vi "ACTION.vi"(8 "error in (no error)":errorcluster, 9 "STEP State":T1, 10 "CORE":refnum<queue>, 11 "Mastering in":refnum<class "Mastering.lvclass">) -> (0 "error out":errorcluster, 3 "Mastering out":refnum<class "Mastering.lvclass">)   [LabVIEW 2014, in "SeqLoop.lvlib" / "STEP Classes.lvlib" / "Mastering.lvclass"]
uses:
  Mastering.lvclass
  TypeDefs/STEP State.ctl
  APIs/Message Queue/Message Cluster.ctl
  Mastering.lvclass/Mastering.ctl
  APIs/Message Queue/Enqueue Message (Array).vi
  APIs/Message Queue/Enqueue Message (Single).vi
  APIs/Message Queue/WINFAS 2 Message Queue.lvlib
  SeqLoop.lvlib
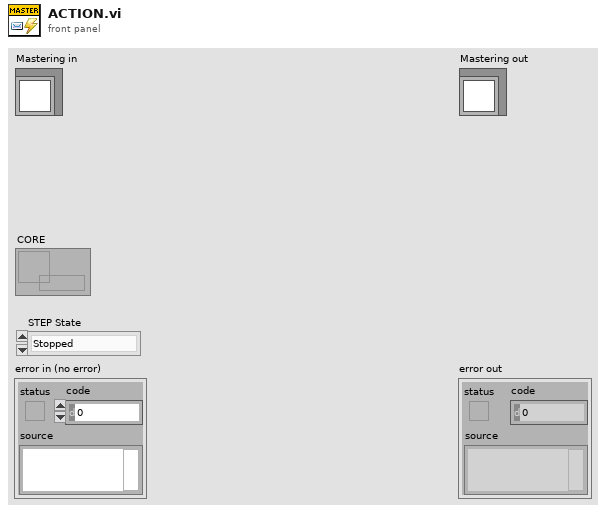
[diagram p1: front panel]
types:
  T1 = typedef "SeqLoop.lvlib/STEP State.ctl" = enum16{"Stopped", "First Call", "Idle...", "Advance OK", "Alarm", "Output Security", "Error"}
  T2 = cluster{"HWSync 1":bool, "HWSync 2":bool, "HWSync 3":bool, "HWSync 4":bool, "HWSync 5":bool}
  T3 = cluster{"MAX(T) or MIN (F)?":bool, "Mastering TDX Index":i32[]}
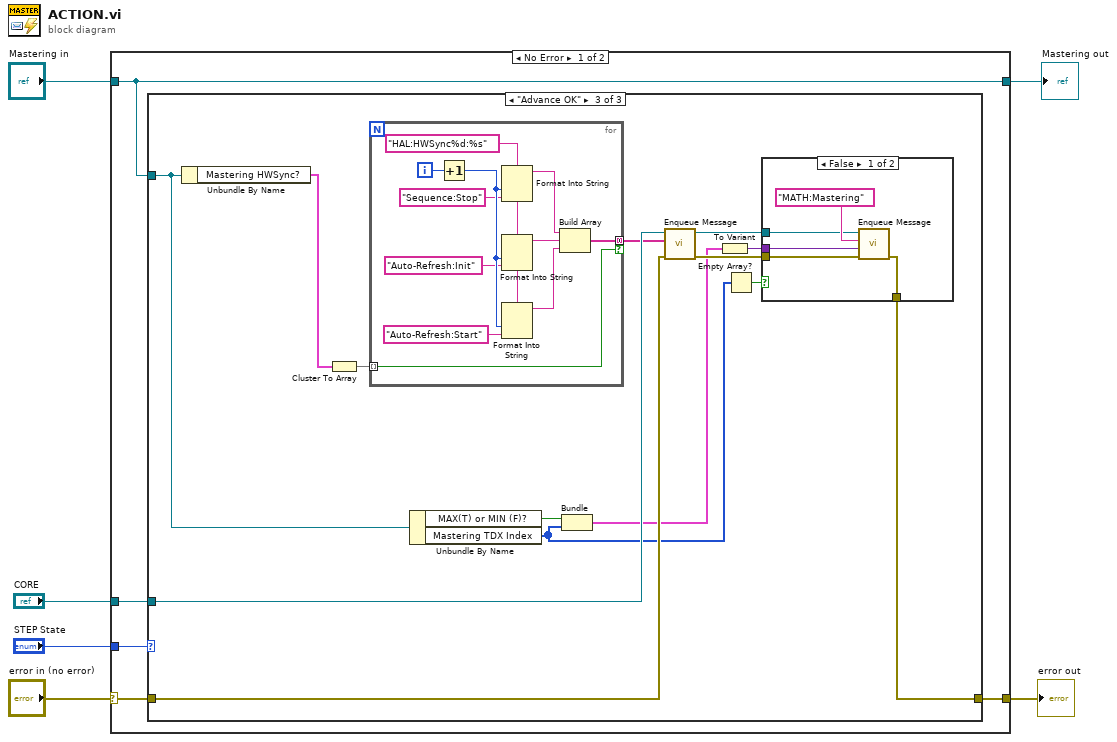
[diagram p0: block diagram]
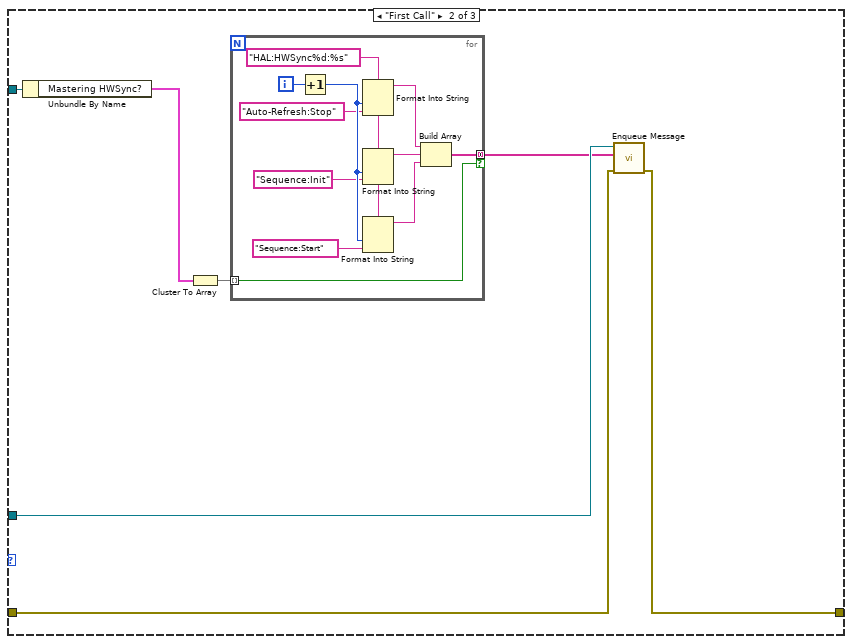
[diagram p3: hidden frame]
diagram:
  n1 = case shown="No Error" "error in (no error)" {
    selector: "error in (no error)" -> [w8 w63]
    tunnel: [w7 w63] -> w2
    tunnel: [w9 w62] -> w1
    tunnel: "Mastering in" -> [w9 w62]
    tunnel: "CORE" -> [w10 _]
    tunnel: "STEP State" -> [w11 _]
    frame No Error {
      n2 = case shown="\"Advance OK\"" w11 {
        tunnel: w10 -> [_ w16 w42]
        tunnel: w9 -> [_ w18 w37]
        tunnel: w8 -> [w12 w15 w41]
        tunnel: [w12 w14 w38] -> w7
        frame Default {
        }
        frame "First Call" {
          n3 = Unbundle By Name(w18) -> ("Mastering HWSync?"=w17:T2)
          n4 = Cluster To Array(cluster=w17) -> (array=w19:bool[])
          n5 = for {
            tunnel: w19 -> [w20] mode=indexing
            tunnel: [w21] -> w13 mode=concatenating if=w20
            i -> [w30]
            w29 = "HAL:HWSync%d:%s" ("format string")
            n6 = Increment(x=w30) -> (x+1=w28:i32)
            n7 = Format Into String(format string=w29, w28, "Auto-Refresh:Stop" ("format string")) -> (resulting string=w24:string)  [unwired: 2 in, 1 out]
            n8 = Format Into String(format string=w29, w28, "Sequence:Init" ("format string")) -> (resulting string=w23:string)  [unwired: 2 in, 1 out]
            n9 = Format Into String(format string=w29, w28, "Sequence:Start" ("format string")) -> (resulting string=w22:string)  [unwired: 2 in, 1 out]
            n10 = Build Array(w24, w23, w22) -> (w21:string[])
          }
          n11 = call-poly "Enqueue Message.vi"("error in (no error)"=w15, "Message Array"=w13, "Message Queue"=w16) -> ("error out"=w14:errorcluster)  [unwired: 7 in, 1 out]
        }
        frame "Advance OK" {
          n12 = Unbundle By Name(w37) -> ("Mastering HWSync?"=w43:T2)
          n13 = Cluster To Array(cluster=w43) -> (array=w44:bool[])
          n14 = for {
            tunnel: w44 -> [w51] mode=indexing
            tunnel: [w52] -> w40 mode=concatenating if=w51
            i -> [w61]
            w60 = "HAL:HWSync%d:%s" ("format string")
            n15 = Increment(x=w61) -> (x+1=w59:i32)
            n16 = Format Into String(format string=w60, w59, "Sequence:Stop" ("format string")) -> (resulting string=w55:string)  [unwired: 2 in, 1 out]
            n17 = Format Into String(format string=w60, w59, "Auto-Refresh:Init" ("format string")) -> (resulting string=w54:string)  [unwired: 2 in, 1 out]
            n18 = Format Into String(format string=w60, w59, "Auto-Refresh:Start" ("format string")) -> (resulting string=w53:string)  [unwired: 2 in, 1 out]
            n19 = Build Array(w55, w54, w53) -> (w52:string[])
          }
          n20 = Unbundle By Name(w37) -> ("MAX(T) or MIN (F)?"=w33:bool, "Mastering TDX Index"=w31:i32[])
          n21 = Bundle("MAX(T) or MIN (F)?"=w33, "Mastering TDX Index"=w31) -> (w34:T3)  [unwired: 1 in]
          n22 = call-poly "Enqueue Message.vi"("error in (no error)"=w41, "Message Array"=w40, "Message Queue"=w42) -> ("error out"=w39:errorcluster, "dup Message Queue"=w36:refnum<queue>)  [unwired: 7 in]
          n23 = To Variant(anything=w34) -> (Variant=w35:variant)
          n24 = Empty Array?(array=w31) -> (empty?=w32:bool)
          n25 = case shown="False" w32 {
            tunnel: w39 -> [w49 w50]
            tunnel: [w48 w50] -> w38
            tunnel: w36 -> [w46 _]
            tunnel: w35 -> [w45 _]
            frame False {
              n26 = call-poly "Enqueue Message.vi"("error in (no error)"=w49, "Message Data"=w45, "Message"="MATH:Mastering" ("format string"), "Message Queue"=w46) -> ("error out"=w48:errorcluster)  [unwired: 6 in, 1 out]
            }
            frame True {
            }
          }
        }
      }
    }
    frame Error {
    }
  }
  "error out" <- w2
  "Mastering out" <- w1
